vi "DmgrEnumDevices.vi"(8 "Error In":errorcluster) -> (0 "Error Out":errorcluster, 2 "Num Devices":i32)   [LabVIEW 2011, in "LVH-Adept.lvlib" / "DMGR.lvlib"]
doc: "Enumerate Devices"
uses:
  DMGR.lvlib
  Type Defs/Error Type.ctl
  LVH-Adept.lvlib
  Resources/dmgr.dll
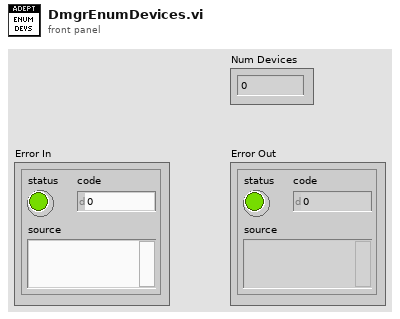
[diagram p1: front panel]
types:
  T1 = typedef "LVH-Adept.lvlib/Error Type.ctl" = enum16{"Unknown Error", "Device Enumeration", "Device Handle", "Device Info"}
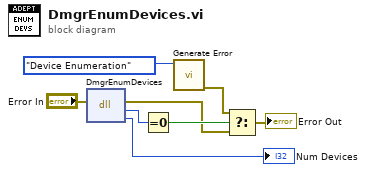
[diagram p0: block diagram]
diagram:
  n1 = dll-call lib="C:/github/labviewhacker/LVH-Adept/LabVIEW/vi.lib/LabVIEW Hacker/Adept/Private/Resources/dmgr.dll" fn="DmgrEnumDevices"(error in="Error In") -> (error out=w1:errorcluster, "Error?"=w6:i8, "pcdvc"=→"Num Devices":i32)  [unwired: 3 in, 1 out]
  n2 = Equal To 0?(x=w6) -> (x = 0?=w5:bool)
  n3 = call "Generate Error.vi"("Error Type"=Error_Type."Device Enumeration") -> ("Error Out"=w2:errorcluster)  [unwired: 10 in]
  n4 = Select(t=w2, s=w5, f=w1) -> (s? t:f=→"Error Out":errorcluster)
